vi "TrapProfile_Execute.vi"(5 "Max Speed (M/S)":dbl format="%20.4f", 6 "TimePeriod":dbl format="%20.4f", 7 "Max Accel":dbl format="%20.4f", 8 "GoalVelocity":dbl format="%20.4f", 9 "GoalPosition":dbl format="%20.4f", 10 "CurrentVelocity":dbl format="%20.4f", 11 "CurrentPosition":dbl format="%20.4f") -> (1 "EstTimeLeft":dbl, 2 "VelocityDmd":dbl, 3 "PositionDmd":dbl)   [LabVIEW 2019, in "Trajectory_Library.lvlib"]
doc: "Convience, single call, LabVIEW function. Creates and calculates a Trapezoid Profile. Call this routine periodically to calculate the newest output for the provided inputs. \n\nOne use of a Trapezoid Profile is to calculate a velocity SP (Setpoint) for a position movement so that the velocity SP creates a trapezoid shape to allow for smoother operation and reduced overshoot. \n \nInputs:\n - Max Speed -- Maximum allowable speed\n - Max Accel -- Maximum allowable acceleration\n - Current Position -- Current position (This could be a measured value.)\n - Current Velocity -- Current velocity (This could be a measured value.)\n - Goal Position -- Deisred final position\n - Goal Velocity -- Desired velocity when goal position is reached. (Might often be zero.)\n - TimePeriod -- Period between calls in seconds.\n\nOutputs:\n - PositionDmd -- Current position demand (This could be used to calculate position error, or used in control.)\n - VelocityDmd -- Current velocity demand. (This could be used as a setpoint to drive an actuator or motor.)\n - EstTimeLeft -- Estimated time remaining until goal is achieved."
uses:
  Trajectory_Library.lvlib
  TrapProfile_Direct.vi
  TrapProfile_ShouldFlipAcceleration.vi
  <vilib>/Rock Robotics/SystemInterfaces/NetworkCommunication/NetComm_UsageReport_report.vi
  Util_LibraryGlobals.vi
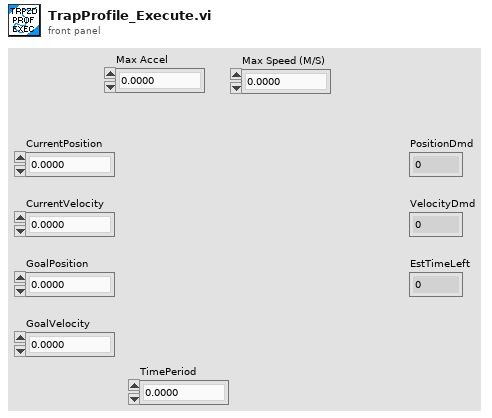
[diagram p1: front panel]
types:
  T1 = typedef "Trajectory_Library.lvlib/TRAPEZOID_PROFILE_STATE.ctl" = cluster{"Position":dbl, "Velocity":dbl}
  T2 = typedef "Trajectory_Library.lvlib/TRAPEZOID_PROFILE_CONSTRAINT.ctl" = cluster{"MaxVelocity":dbl, "MaxAcceleration":dbl}
  T3 = typedef "Trajectory_Library.lvlib/TRAPEZOID_PROFILE.ctl" = cluster{"EndAccel":dbl, "EndFullSpeed":dbl, "EndDecel":dbl, "Direction":i32, "Constraints":T2, "Initial":T1, "Goal":T1}
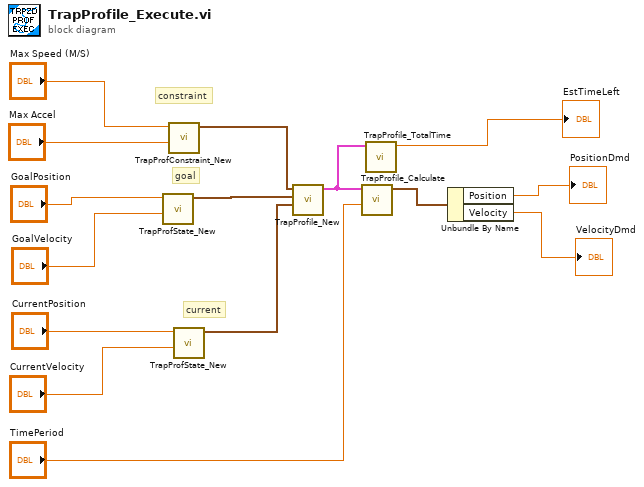
[diagram p0: block diagram]
diagram:
  # "current"
  # "goal"
  # "constraint"
  n1 = call "TrapProfState_New.vi"("Velocity"="GoalVelocity", "Position"="GoalPosition") -> ("TRAPEZOID_PROFILE_STATE"=w15:T1)  [unwired: 9 in]
  n2 = call "TrapProfConstraint_New.vi"("Max Accel"="Max Accel", "Max Speed (M/S)"="Max Speed (M/S)") -> ("TRAPEZOID_PROFILE_CONSTRAINT"=w14:T2)  [unwired: 9 in]
  n3 = call "TrapProfState_New.vi"("Velocity"="CurrentVelocity", "Position"="CurrentPosition") -> ("TRAPEZOID_PROFILE_STATE"=w12:T1)  [unwired: 9 in]
  n4 = call "TrapProfile_New.vi"("Initial"=w12, "Goal"=w15, "Constraints"=w14) -> ("TRAPEZOID_PROFILE"=w13:T3)  [unwired: 8 in]
  n5 = call "TrapProfile_Calculate.vi"("Time"="TimePeriod", "TRAPEZOID_PROFILE"=w13) -> ("State"=w10:T1)  [unwired: 9 in]
  n6 = call "TrapProfile_TotalTime.vi"("TRAPEZOID_PROFILE"=w13) -> ("TotalTime"=→"EstTimeLeft":dbl)  [unwired: 10 in]
  n7 = Unbundle By Name(w10) -> ("Position"=→"PositionDmd":dbl, "Velocity"=→"VelocityDmd":dbl)
